vi "Slave on Desktop（RTU）.vi"() -> ()   [LabVIEW 2017]
doc: "Demonstrates how to use Modbus functions to create a slave listening to a specific TCP port. It shows an interactive UI to allow users read and write the coils on a virtual slave device. Users can also get the count of masters connected to this slave."
uses:
  <vilib>/Modbus/slave/Create Slave Instance (Serial).vi
  <vilib>/Modbus/slave/Modbus Slave.lvclass
panel:
  out "register values":u16[](array[numeric])
  in  "holding register values":u16[](array[numeric])
  in  "baud rate (9600)":u32=9600
  in  "Read Count":u16=10
  in  "Stop":bool
  in  "Read":bool
  in  "Write":bool
  # "Write Operation"
  # "Read Operation"
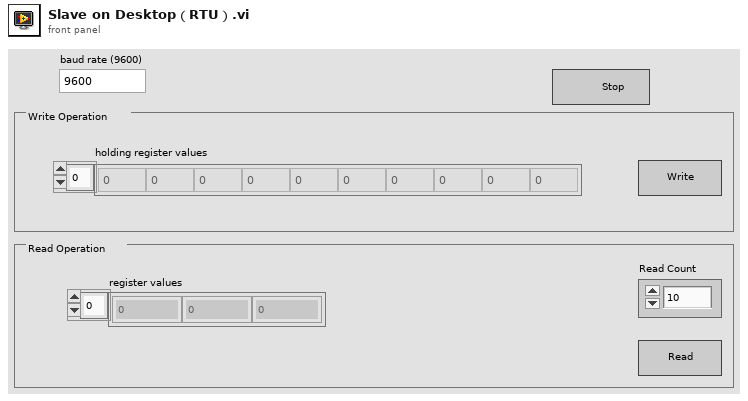
[diagram p1: front panel]
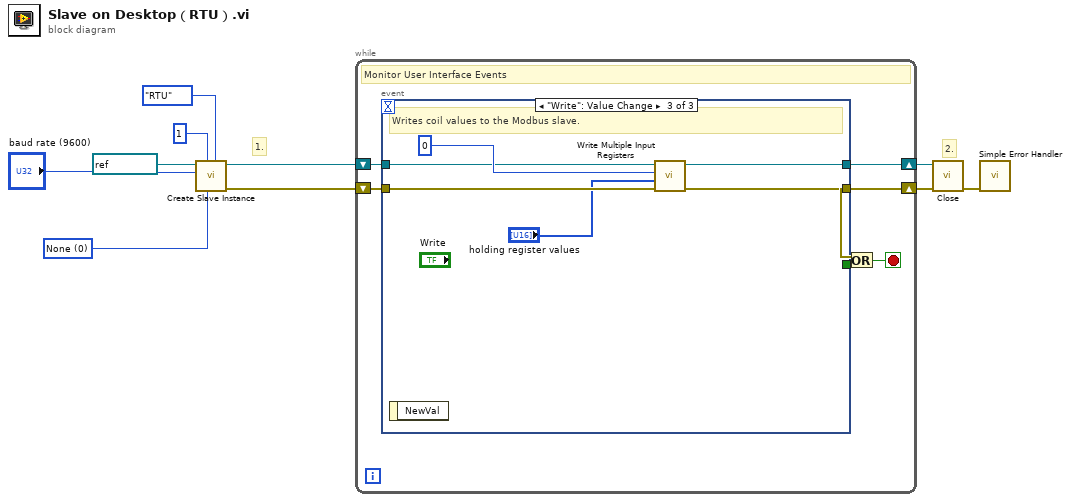
[diagram p0: block diagram]
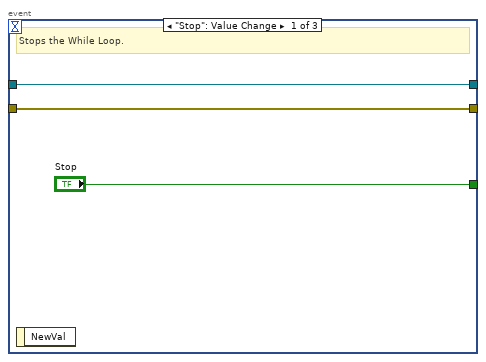
[diagram p2: hidden frame]
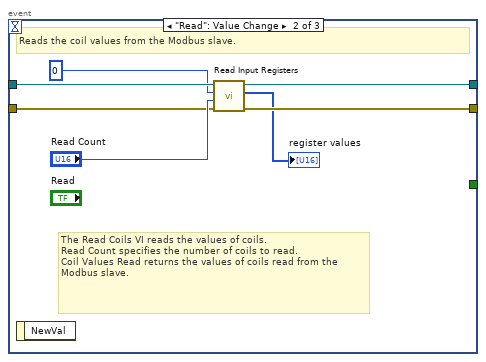
[diagram p3: hidden frame]
diagram:
  w1 = u16 0 items=["None", "Odd", "Even"] ("parity (Even)")
  # "2."
  # "1."
  n1 = call-poly <vilib>:"Create Slave Instance.vi"("serial type"=enum16{"RTU", "ASCII"}."RTU", "parity (Even)"=w1, "unit ID"=u8 1, "baud rate (9600)"="baud rate (9600)", "VISA resource name"=refnum<visa-resource-name> "COM3") -> ("error out"=w9:errorcluster, "serial slave instance"=w10:refnum<class "Modbus Slave.lvclass">)  [unwired: 5 in]
  n2 = while {
    shift-right: [w15] -> w7
    shift-left: w10 -> [w16]
    shift-right: [w13] -> w8
    shift-left: w9 -> [w14]
    stop <- w11 stop-if-true
    # "Monitor User Interface Events"
    n3 = event shown="[2] \"Write\": Value Change" {
      selector: _ -> [_ _ _]
      dyn-events: _ -> [_ _ _]
      timeout: _ -> [_ _ _]
      tunnel: ["Stop" _ _] -> w12
      tunnel: w16 -> [w18 w26 w31]
      tunnel: [w18 w25 w30] -> w15
      tunnel: w14 -> [w19 w22 w29]
      tunnel: [w19 w21 w28] -> w13
      event "Stop": Value Change {
        # "Stops the While Loop."
        n4 = event-data() -> ()  [unwired: 1 in, 1 out]
      }
      event "Read": Value Change {
        # "The Read Coils VI reads the values of coils.\nRead Count specifies the number of coils to read.\nCoil Values Read returns the values of coils read from the Modbus slave."
        # "Reads the coil values from the Modbus slave."
        n5 = event-data() -> ()  [unwired: 1 in, 1 out]
        n6 = call-dynamic "Read Input Registers.vi"("error in (no error)"=w22, "number of input registers"="Read Count", "starting address"=u16 0, "Modbus slave in"=w26) -> ("error out"=w21:errorcluster, "register values"=→"register values":u16[], "Modbus slave out"=w25:refnum<class "Modbus Slave.lvclass">)  [unwired: 5 in]
      }
      event "Write": Value Change {
        # "Writes coil values to the Modbus slave."
        n7 = event-data() -> ()  [unwired: 1 in, 1 out]
        n8 = call-dynamic "Write Multiple Input Registers.vi"("error in (no error)"=w29, "input register values"="holding register values", "starting address"=u16 0, "Modbus slave in"=w31) -> ("error out"=w28:errorcluster, "Modbus slave out"=w30:refnum<class "Modbus Slave.lvclass">)  [unwired: 6 in]
      }
    }
    n9 = Or(x=w13, y=w12) -> (x .or. y?=w11:bool)
  }
  n10 = call-dynamic "Close.vi"("error in (no error)"=w8, "Modbus slave in"=w7) -> ("error out"=w6:errorcluster)  [unwired: 9 in]
  n11 = call <vilib>:"Simple Error Handler.vi"("error in (no error)"=w6) -> ()  [unwired: 4 in, 5 out]
